vi "Scroller_FGGA_Pump_test_server.vi"() -> ()   [LabVIEW 2014]
uses:
  <vilib>/NI/STM/SubVIs/MetaDataElement.ctl
  <vilib>/Platform/TimedLoop/XDataNode/timing_clust.ctl
  <vilib>/Platform/TimedLoop/XDataNode/nitl_modes.ctl
  <vilib>/Platform/TimedLoop/XDataNode/wakeup.ctl
  <vilib>/NI/STM/TCP/Write Meta Data (TCP Ref).vi
  <vilib>/NI/STM/TCP/Get Connection Reference (TCP).vi
  <vilib>/NI/STM/TCP/Write Meta Data (TCP Clst).vi
  <vilib>/NI/STM/TCP/Write Message (TCP).vi
  <vilib>/platform/TimedLoop/XDataNode/XDataNode.xnode
  <vilib>/Platform/TimedLoop/XDataNode/XDNodeRunTimeDep.lvlib
  <vilib>/NI/STM/NI STM.lvlib
panel:
  out "error out":errorcluster
  out "appended array":string[](array[string])
  in  "Array 2":string[](array[string])
  in  "Standby Speed threshold":u32(slide) scale=66.0..100.0
  in  "Normal Speed threshold":u32(slide) scale=50.0..100.0
  out "running?":bool
  in  "Set AutoRun":bool
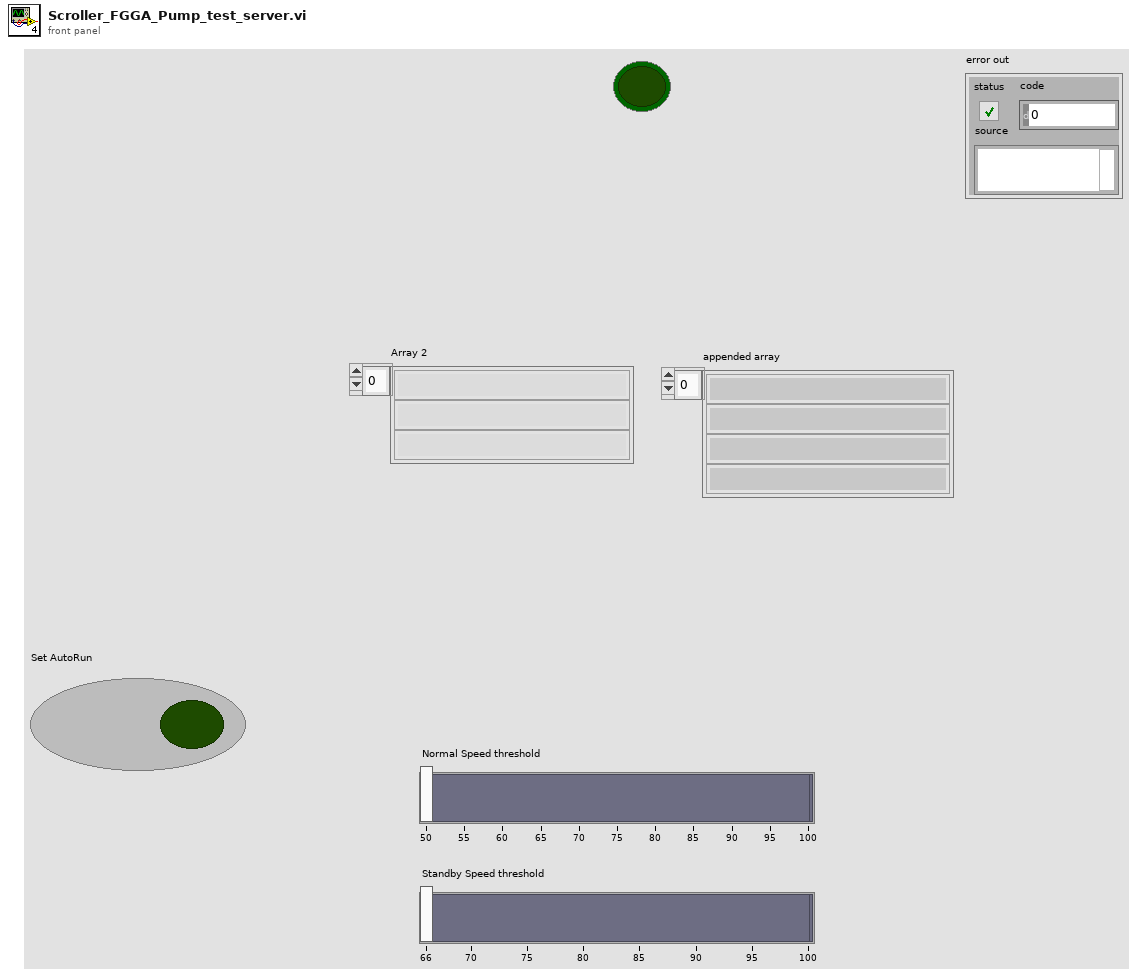
[diagram p1: front panel]
types:
  T1 = typedef "XDNodeRunTimeDep.lvlib/timing_clust.ctl" = cluster{"Expected End [f-1]":u64, "Actual End [f-1]":u64, "Finished Late? [f-1]":bool, "Expected End [i-1]":u64, "Actual End [i-1]":u64, "Finished Late? [i-1]":bool, "Expected Start [i]":u64, "Actual Start [i]":u64, "Expected Start [f]":u64, "Actual Start [f]":u64, "Source Name":string, "Structure Name":string, "Period":i64, "Deadline":i64, "Offset":i64, "Start":i64, "Priority":i32, "Timeout":i32, "Mode":T2, "Wakeup Reason":T3, "Error":errorcluster, "Source Type":string, "Secondary Source Type":string, "Global End Time":u64, "Global Start Time":u64, "Frame Duration":u64, "Iteration Duration":u64, "Assigned CPU":i32, "I/O Scan Engine Mode":u32}
  T2 = typedef "XDNodeRunTimeDep.lvlib/nitl_modes.ctl" = enum32{"No Change", "Process missed periods, maintain original phase", "Discard missed periods, maintain original phase", "Process missed periods, ignore original phase", "Discard missed periods, ignore original phase"}
  T3 = typedef "XDNodeRunTimeDep.lvlib/wakeup.ctl" = enum32{"Normal", "Aborted", "Asynchronous wakeup", "Timing source error", "Timed loop error", "Timeout"}
  T4 = typedef "NI STM.lvlib/MetaDataElement.ctl" = string
  T5 = typedef "NI STM.lvlib/TCP Connection Info.ctl" = cluster{"connection ID":refnum<k5>, "meta data":T4[]}
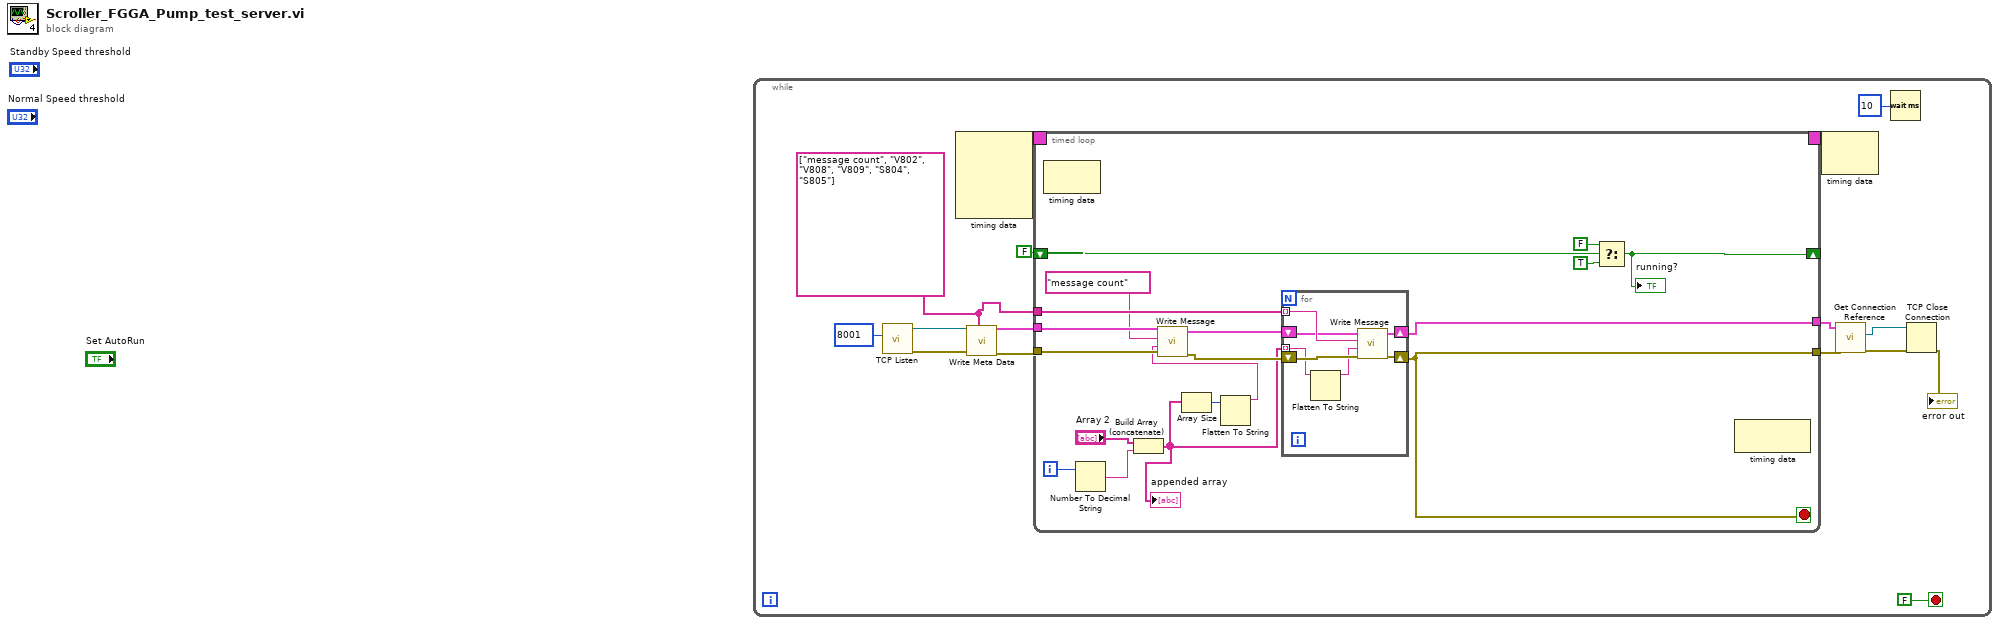
[diagram p0: block diagram]
diagram:
  n1 = while {
    stop <- FALSE stop-if-true
    w1 = T4[] ["message count", "V802", "V808", "V809", "S804", "S805"] ("meta data")
    n2 = call <vilib>:"TCP Listen.vi"("port"=u16 8001) -> ("error out"=w9:errorcluster, "connection ID"=w10:refnum<k5>)  [unwired: 6 in, 3 out]
    n3 = node-c288() -> (w16:T1)  [unwired: 4 in]
    n4 = call-poly <vilib>:"Write Meta Data.vi"("meta data"=w1, "error in"=w9, "connection ID"=w10) -> ("error out"=w8:errorcluster, "connection info out"=w7:T5)  [unwired: 2 in, 5 out]
    n5 = timed-loop {
      shift-right: [w31] -> _
      shift-left: FALSE -> [w34]
      timing: w16 -> [_]
      timing-out: [_] -> w15
      tunnel: w7 -> [w24]
      tunnel: w8 -> [w23]
      tunnel: w1 -> [w27]
      tunnel: [w26] -> w4
      tunnel: [w25] -> w5
      i -> [w30]
      stop <- w26 stop-if-true
      n6 = node-c288() -> ()  [unwired: 1 in, 1 out]
      n7 = Number To Decimal String(number=w30) -> (decimal integer string=w28:string)  [unwired: 1 in]
      n8 = Build Array (concatenate)("Array 2", w28) -> (w19:string[])
      "appended array" <- w19
      n9 = Array Size(array=w19) -> (size(s)=w18:i32)
      n10 = Flatten To String(anything=w18) -> (data string=w17:string)  [unwired: 1 in, 4 out]
      n11 = call-poly <vilib>:"Write Message.vi"("error in"=w23, "data"=w17, "name"="message count", "connection info in"=w24) -> ("error out"=w22:errorcluster, "connection info out"=w21:T5)  [unwired: 1 in, 5 out]
      n12 = for {
        tunnel: w19 -> [w36] mode=indexing
        tunnel: w27 -> [w41] mode=indexing
        shift-right: [w37] -> w25
        shift-left: w21 -> [w40]
        shift-right: [w38] -> w26
        shift-left: w22 -> [w39]
        n13 = Flatten To String(anything=w36) -> (data string=w35:string)  [unwired: 1 in, 4 out]
        n14 = call-poly <vilib>:"Write Message.vi"("error in"=w39, "data"=w35, "name"=w41, "connection info in"=w40) -> ("error out"=w38:errorcluster, "connection info out"=w37:T5)  [unwired: 1 in, 5 out]
      }
      n15 = Select(t=FALSE, s=w34, f=TRUE) -> (s? t:f=w31:bool)
      "running?" <- w31
      n16 = node-c288() -> ()  [unwired: 1 in, 1 out]
    }
    n17 = node-c288(w15) -> ()  [unwired: 1 out]
    n18 = call-poly <vilib>:"Get Connection Reference.vi"("error in"=w4, "connection info in"=w5) -> ("error out"=w6:errorcluster, "connection ID out"=w3:refnum<k5>)  [unwired: 8 out]
    n19 = Wait (ms)(milliseconds to wait=u32 10) -> ()  [unwired: 1 out]
    n20 = TCP Close Connection(connection ID=w3, error in (no error)=w6) -> (error out=→"error out":errorcluster)  [unwired: 2 out]
  }
